vi "Remove DG by DGNr.vi"(8 "error in (no error)":errorcluster, 10 "DG Nr.":i32=1 min=1, 11 "BME_DG_System in":refnum<class "BME_DG_System.lvclass">) -> (0 "error out":errorcluster, 1 "found?":bool, 2 "Deleted DG":refnum<class "BME_DG_Base.lvclass">, 3 "BME_DG_System out":refnum<class "BME_DG_System.lvclass">)   [LabVIEW 2009, in "POLARIS BME DG.lvlib" / "BME_DG_System.lvclass"]
uses:
  BME_DG_System.lvclass
  BME_DG_Base/BME_DG_Base.lvclass
  BME_DG_System.lvclass/BME_DG_System.ctl
  POLARIS BME DG.lvlib
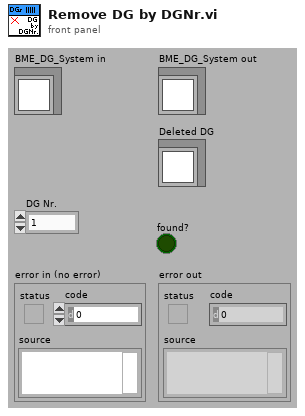
[diagram p1: front panel]
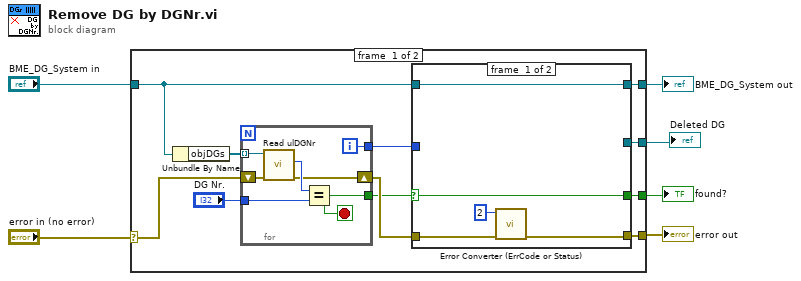
[diagram p0: block diagram]
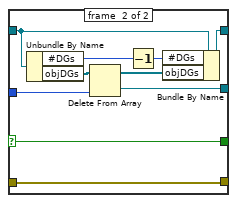
[diagram p2: hidden frame]
diagram:
  n1 = case shown="No Error" "error in (no error)" {
    selector: "error in (no error)" -> [w14 w40]
    tunnel: [w13 w40] -> w5
    tunnel: [w8 w41] -> w3
    tunnel: "BME_DG_System in" -> [w9 w41]
    tunnel: [w11 _] -> w2
    tunnel: [w7 _] -> w1
    frame #0 {
      n2 = Unbundle By Name(w9) -> ("objDGs"=w17:refnum<class "BME_DG_Base.lvclass">[])
      n3 = for {
        tunnel: w17 -> [w39] mode=indexing
        tunnel: "DG Nr." -> [w37]
        tunnel: [w36] -> w12
        shift-right: [w34] -> w15
        shift-left: w14 -> [w35]
        tunnel: [w33] -> w10
        i -> [w33]
        stop <- w36 stop-if-true
        n4 = call-dynamic "Read ulDGNr.vi"("error in (no error)"=w35, "BME_DG_Base in"=w39) -> ("error out"=w34:errorcluster, "ulDGNr"=w38:u32)  [unwired: 6 in, 2 out]
        n5 = Equal?(x=w38, y=w37) -> (x = y?=w36:bool)
      }
      n6 = case shown="True" w12 {
        selector: w12 -> [w19 w31]
        tunnel: w15 -> [w21 w32]
        tunnel: [w20 w32] -> w13
        tunnel: [w19 w31] -> w11
        tunnel: w10 -> [_ w30]
        tunnel: w9 -> [w18 w27]
        tunnel: [w18 w29] -> w8
        tunnel: [_ w23] -> w7
        frame #0 {
          n7 = call "Error Converter (ErrCode or Status).vi"("error in (no error)"=w21, "error code"=2) -> ("error out"=w20:errorcluster)  [unwired: 9 in]
        }
        frame #1 {
          n8 = Unbundle By Name(w27) -> ("#DGs"=w25:i32, "objDGs"=w26:refnum<class "BME_DG_Base.lvclass">[])
          n9 = Delete From Array(array=w26, index=w30) -> (deleted portion=w23:refnum<class "BME_DG_Base.lvclass">, array with subset deleted=w28:refnum<class "BME_DG_Base.lvclass">[])  [unwired: 1 in]
          n10 = Decrement(x=w25) -> (x-1=w24:i32)
          n11 = Bundle By Name(cluster=w27, "#DGs"=w24, "objDGs"=w28) -> (w29:refnum<class "BME_DG_System.lvclass">)
        }
      }
    }
    frame #1 {
    }
  }
  "error out" <- w5
  "BME_DG_System out" <- w3
  "found?" <- w2
  "Deleted DG" <- w1
